vi "BRig_dataExp_Cue2_1A_Prob.vi"() -> (2 "output_Cue2_1A_Prob":i32)   [LabVIEW 2014]
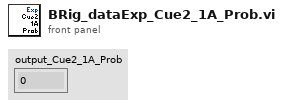
[diagram p1: front panel]
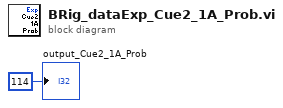
[diagram p0: block diagram]
diagram:
  "output_Cue2_1A_Prob" <- 114 ("output_iBlock")
